vi "parse_bool_roslv.vi"   [LabVIEW 2014]
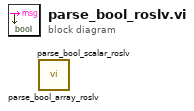
[diagram p0: block diagram]
diagram:
  n1 = call "parse_bool_array_roslv.vi"() -> ()  [unwired: 5 in, 3 out]
  n2 = call "parse_bool_scalar_roslv.vi"() -> ()  [unwired: 5 in, 3 out]
